vi "Get Current Available GU.vi"(8 "error in":errorcluster, 11 "Config Data":T1(array[cluster])) -> (0 "error out":errorcluster, 2 "All Available GU":i32[](array[numeric]), 3 "Config Data dup":T1(array[cluster]))   [LabVIEW 2020, in "GUCalibration2.lvlib"]
uses:
  GUCalibration2.lvlib
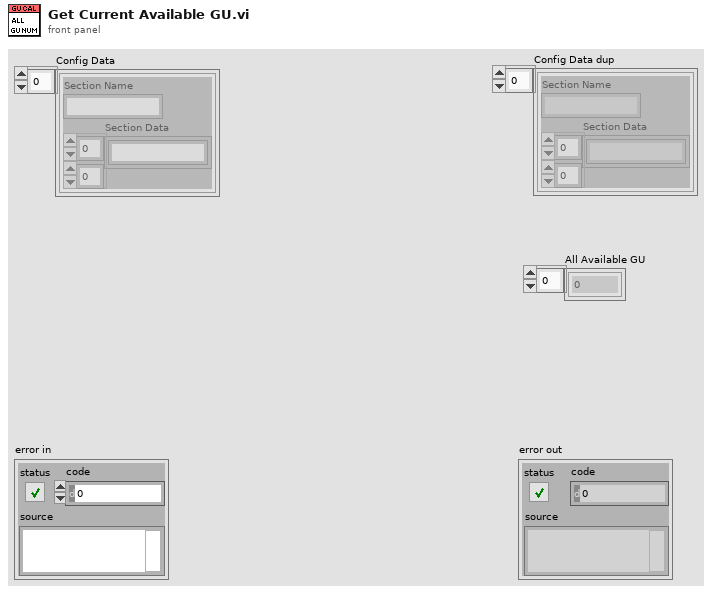
[diagram p1: front panel]
types:
  T1 = cluster{"Section Name":string, "Section Data":string[][]}[]
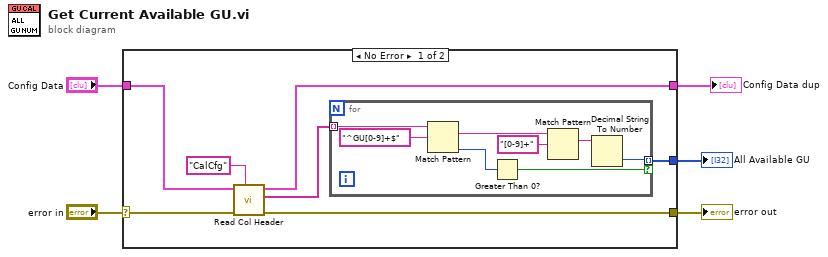
[diagram p0: block diagram]
diagram:
  n1 = case shown="No Error" "error in" {
    selector: "error in" -> [w7 w21]
    tunnel: "Config Data" -> [w11 w22]
    tunnel: [w9 _] -> w4
    tunnel: [w8 w21] -> w3
    tunnel: [w6 w22] -> w1
    frame No Error {
      n2 = call "Read Col Header.vi"("Section Name"="CalCfg", "error in (no error)"=w7, "Config Data"=w11) -> ("error out"=w8:errorcluster, "Column Header"=w10:string[], "Config Data dup"=w6:T1)  [unwired: 4 in, 2 out]
      n3 = for {
        tunnel: w10 -> [w15] mode=indexing
        tunnel: [w14] -> w9 mode=indexing if=w13
        n4 = Match Pattern(string=w15, regular expression="^GU[0-9]+$") -> (match substring=w18:string, offset past match=w19:i32)  [unwired: 1 in, 2 out]
        n5 = Greater Than 0?(x=w19) -> (x > 0?=w13:bool)
        n6 = Match Pattern(string=w18, regular expression="[0-9]+") -> (match substring=w16:string)  [unwired: 1 in, 3 out]
        n7 = Decimal String To Number(string=w16) -> (number=w14:i32)  [unwired: 2 in, 1 out]
      }
    }
    frame Error {
    }
  }
  "All Available GU" <- w4
  "error out" <- w3
  "Config Data dup" <- w1
